vi "SR-M_Load-Mission.vi"(11 "Mission In in":T1[](array[typedef]) {"GPS Longitude" format="%.6g"; "GPS Latitude" format="%.6g"}) -> (3 "Mission In out":T1[](array[typedef]) {"GPS Longitude" format="%.6g"; "GPS Latitude" format="%.6g"})   [LabVIEW 2015, in "Shore Library.lvlib"]
uses:
  Shore Library.lvlib
  RDS Mission Controller Actor/MissionOp.ctl
  RDS Mission Controller Actor/RDS Mission Controller Actor.lvlib
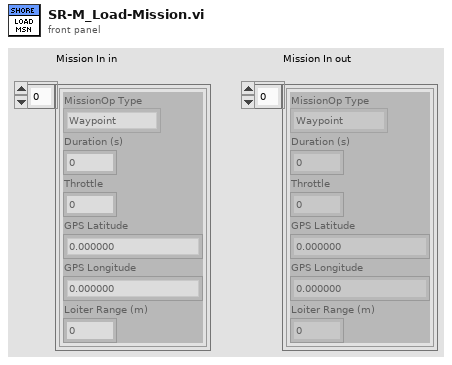
[diagram p1: front panel]
types:
  T1 = typedef "RDS Mission Controller Actor.lvlib/MissionOp.ctl" = cluster{"MissionOp Type":enum16{"Waypoint", "Loiter", "Wait", "Deploy AIP", "Stow AIP"}, "Duration (s)":u16, "Throttle":i16, "GPS Latitude":dbl, "GPS Longitude":dbl, "Loiter Range (m)":u16}
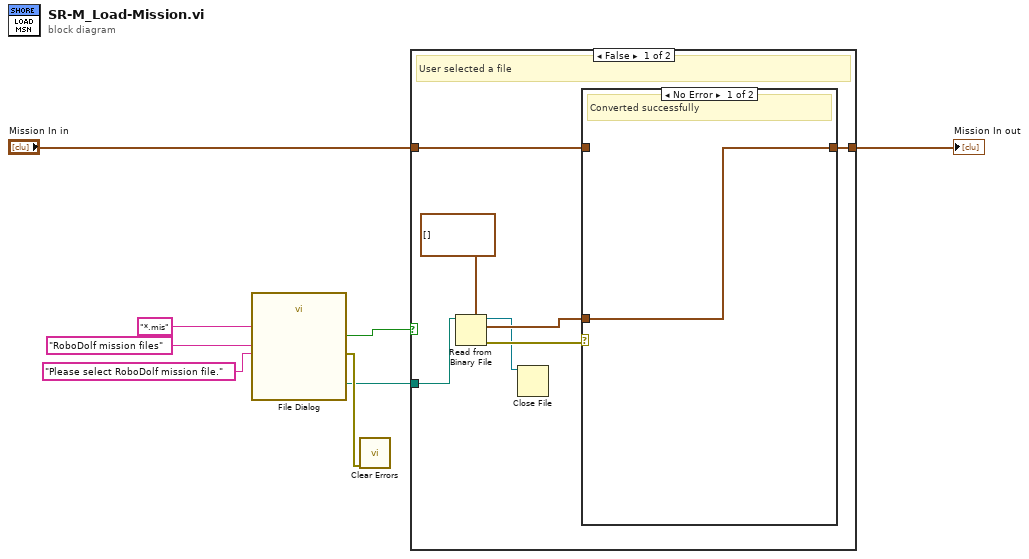
[diagram p0: block diagram]
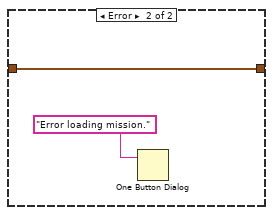
[diagram p2: hidden frame]
diagram:
  n1 = call "File Dialog"("prompt"="Please select RoboDolf mission file." ("prompt (Open existing file)"), "pattern (all files)"="*.mis", "pattern label"="RoboDolf mission files") -> ("selected path"=w3:path, "cancelled"=w4:bool, "error out"=w8:errorcluster)  [unwired: 9 in, 1 out]
  n2 = call <vilib>:"Clear Errors.vi"("error in (no error)"=w8) -> ()  [unwired: 5 in, 2 out]
  n3 = case shown="False" w4 {
    tunnel: "Mission In in" -> [w15 w19]
    tunnel: [w14 w19] -> w2
    tunnel: w3 -> [w10 _]
    frame False {
      # "User selected a file"
      n4 = Read from Binary File(5:T1[] [] ("Mission In"), 11:w10) -> (0:w11:errorcluster, 2:w12:T1[], 3:w9:refnum<file>)  [unwired: 4 in, 1 out]
      n5 = Close File(refnum=w9) -> ()  [unwired: 1 in, 2 out]
      n6 = case shown="No Error" w11 {
        tunnel: w12 -> [w16 _]
        tunnel: [w16 w18] -> w14
        tunnel: w15 -> [_ w18]
        frame No Error {
          # "Converted successfully"
        }
        frame Error {
          n7 = One Button Dialog(message="Error loading mission.") -> ()  [unwired: 1 in, 1 out]
        }
      }
    }
    frame True {
    }
  }
  "Mission In out" <- w2
